vi "HardWare Globals.vi"() -> ()   [LabVIEW 2016]
panel:
  in  "ProductID":string
  out "AutoSelect?":bool
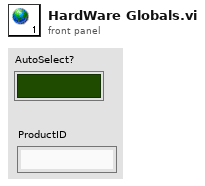
[diagram p1: front panel]
diagram:
